vi "Timestamp_Anlysis_with_Calibration.vi"(8 "error in (no error)":errorcluster, 9 "Calibrate?":bool, 10 "Warmup iterations":i32=10, 11 "Timestamp Array":u64[](array[numeric])) -> (0 "error out":errorcluster, 1 "execution histogram":T1(graph), 2 "execution times (uS)":dbl[](graph), 3 "max jitter (uS)":dbl format="%.2f", 4 "standard deviation (uS)":dbl format="%.2f", 5 "mean time (uS)":dbl format="%.2f", 6 "Max Jitter Point":cluster{"X":dbl, "Y":dbl})   [LabVIEW 2014]
uses:
  Program Files (x86)/National Instruments/LabVIEW 2014/Targets/NI/RT/vi.lib/NI_Real-Time Target Support.lvlib
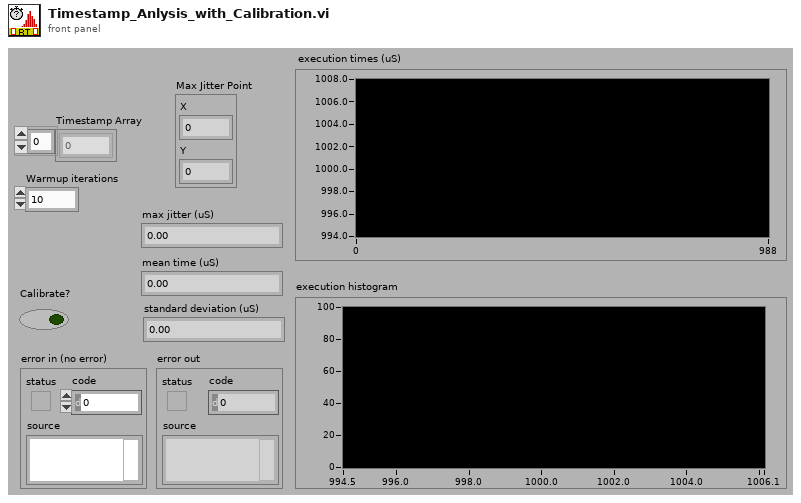
[diagram p1: front panel]
types:
  T1 = cluster{"X Values":dbl[], "Histogram: h(x)":i32[]}
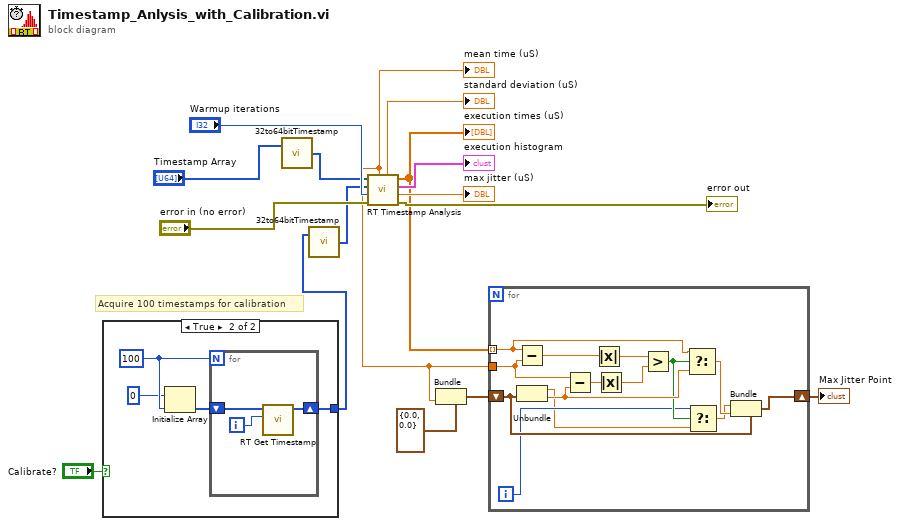
[diagram p0: block diagram]
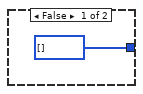
[diagram p2: hidden frame]
diagram:
  # "Acquire 100 timestamps for calibration"
  n1 = case shown="True" "Calibrate?" {
    tunnel: [u64[] [] w21] -> w2
    frame False {
    }
    frame True {
      w19 = 100
      n2 = Initialize Array(u64 0, w19) -> (w20:u64[])
      n3 = for {
        N: w19 -> [_]
        shift-right: [w22] -> w21
        shift-left: w20 -> [w23]
        i -> [w24]
        n4 = call "RT Get Timestamp.vi"("iteration"=w24, "timestamp array in"=w23) -> ("timestamp array out"=w22:u64[])  [unwired: 8 in, 1 out]
      }
    }
  }
  n5 = call "32to64bitTimestamp.vi"("Timestamps In"="Timestamp Array") -> ("Timestamps Out"=w3:u64[])  [unwired: 1 in]
  n6 = call "32to64bitTimestamp.vi"("Timestamps In"=w2) -> ("Timestamps Out"=w1:u64[])  [unwired: 1 in]
  n7 = call "RT Timestamp Analysis.vi"("error in (no error)"="error in (no error)", "warmup iterations"="Warmup iterations", "calibration array"=w1, "timestamp array"=w3) -> ("error out"=→"error out":errorcluster, "max jitter (uS)"=→"max jitter (uS)":dbl, "execution histogram"=→"execution histogram":T1, "execution times (uS)"=w9:dbl[], "standard deviation (uS)"=→"standard deviation (uS)":dbl, "mean time (uS)"=w6:dbl)  [unwired: 2 in]
  "execution times (uS)" <- w9
  "mean time (uS)" <- w6
  n8 = Bundle(cluster=cluster{"X":dbl, "Y":dbl} {"X"=0.0, "Y"=0.0}, "Y"=w6) -> (w5:cluster{"X":dbl, "Y":dbl})  [unwired: 1 in]
  n9 = for {
    tunnel: w9 -> [w32] mode=indexing
    shift-right: [w33] -> w8
    shift-left: w5 -> [w35]
    tunnel: w6 -> [w31]
    i -> [w26]
    n10 = Subtract(x=w32, y=w31) -> (x-y=w38:dbl)
    n11 = Unbundle(w35) -> ("X"=w25:dbl, "Y"=w29:dbl)
    n12 = Subtract(x=w31, y=w29) -> (x-y=w30:dbl)
    n13 = Absolute Value(x=w38) -> (abs(x)=w37:dbl)
    n14 = Absolute Value(x=w30) -> (abs(x)=w36:dbl)
    n15 = Greater?(x=w37, y=w36) -> (0:w28:bool)
    n16 = Select(t=w32, s=w28, f=w29) -> (s? t:f=w34:dbl)
    n17 = Select(t=w26, s=w28, f=w25) -> (s? t:f=w27:dbl)
    n18 = Bundle(cluster=w35, "X"=w27, "Y"=w34) -> (w33:cluster{"X":dbl, "Y":dbl})
  }
  "Max Jitter Point" <- w8
